vi "质控数据存储(子VI).vi"(4 "CODMn":refnum<vi>, 6 "总磷":refnum<vi>, 7 "CODCr":refnum<vi>, 10 "氨氮":refnum<vi>, 11 "总氮":refnum<vi>) -> ()   [LabVIEW 2016, in "质控单元.lvlib"]
uses:
  <vilib>/ptbypt/NI_PtbyPt.lvlib
panel:
  out "columns":string[](array[string])
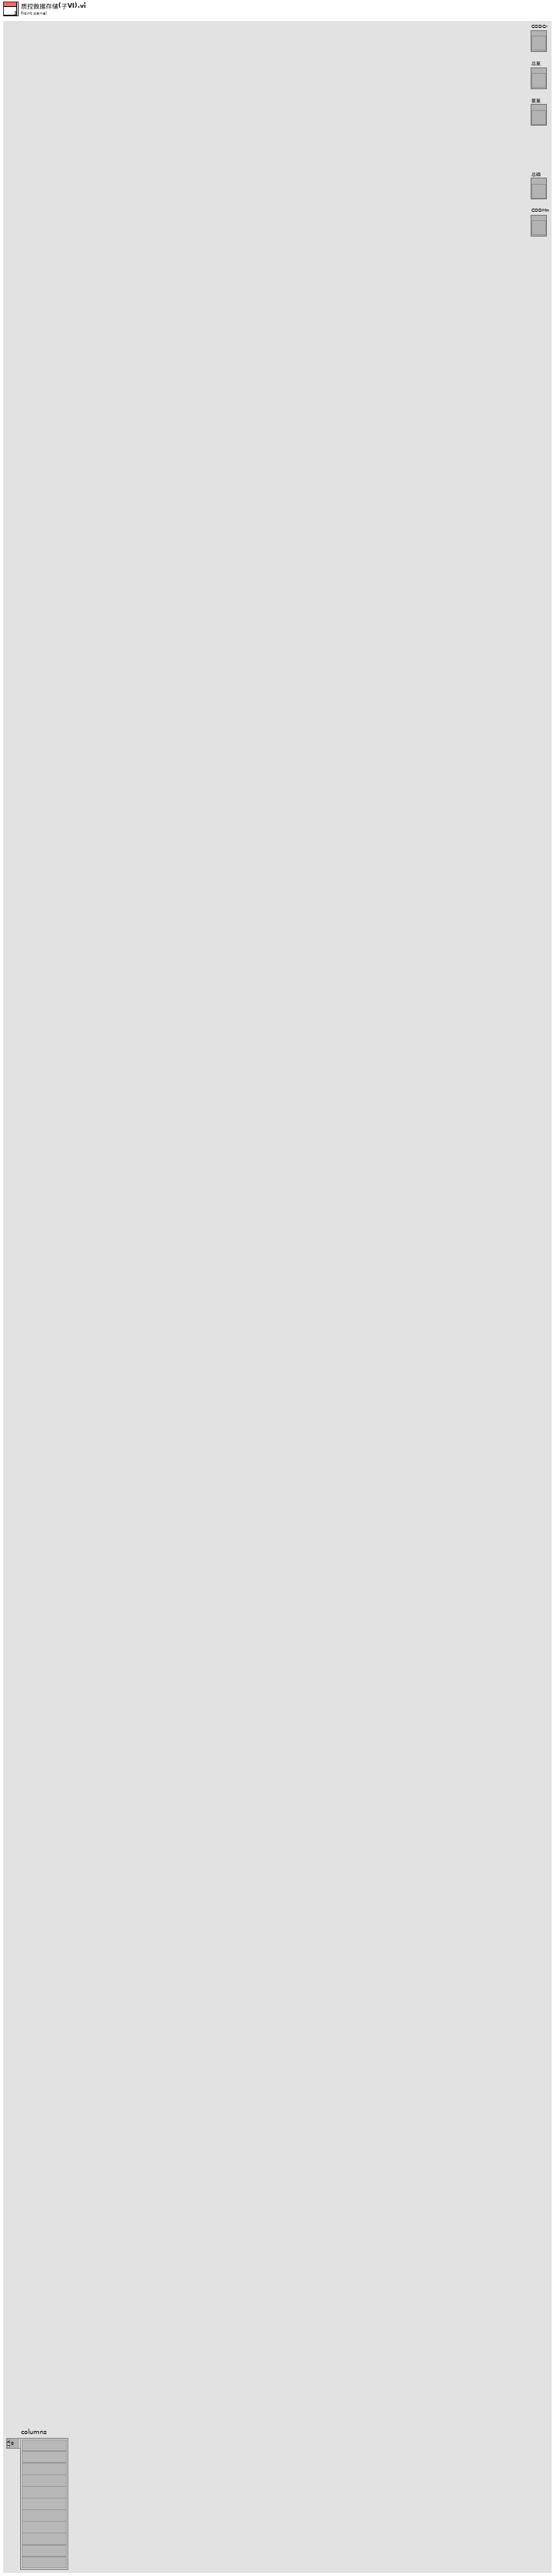
[diagram p1: front panel]
types:
  T1 = cluster{"时间":timestamp, "参数":string, "数据类型":string, "加标前水样测试时间":timestamp, "加标前水样浓度值（mg/L)":sgl, "加标后水样浓度值（mg/L)":sgl, "加标母液浓度值（mg/L)":sgl, "加标体积":dbl, "加标水杯定容体积":dbl, "加标回收率":dbl}
  T2 = cluster{"因子编码":u32, "单位":u16, "标样参考值":sgl, "水样数据时间":timestamp, "水样实测值":sgl, "水样数据标识":string, "标样数据时间":timestamp, "标样实测值":sgl, "标样数据标识":string, "空白数据时间":timestamp, "空白实测值":sgl, "空白数据标识":string, "零点核查数据时间":timestamp, "零点核查实测值":sgl, "零点核查数据标识":string, "跨度核查数据时间":timestamp, "跨度核查实测值":sgl, "跨度核查数据标识":string, "加标回收数据时间":timestamp, "加标回收实测值":sgl, "加标回收数据标识":string, "平行样数据时间":timestamp, "平行样实测值":sgl, "平行样数据标识":string}
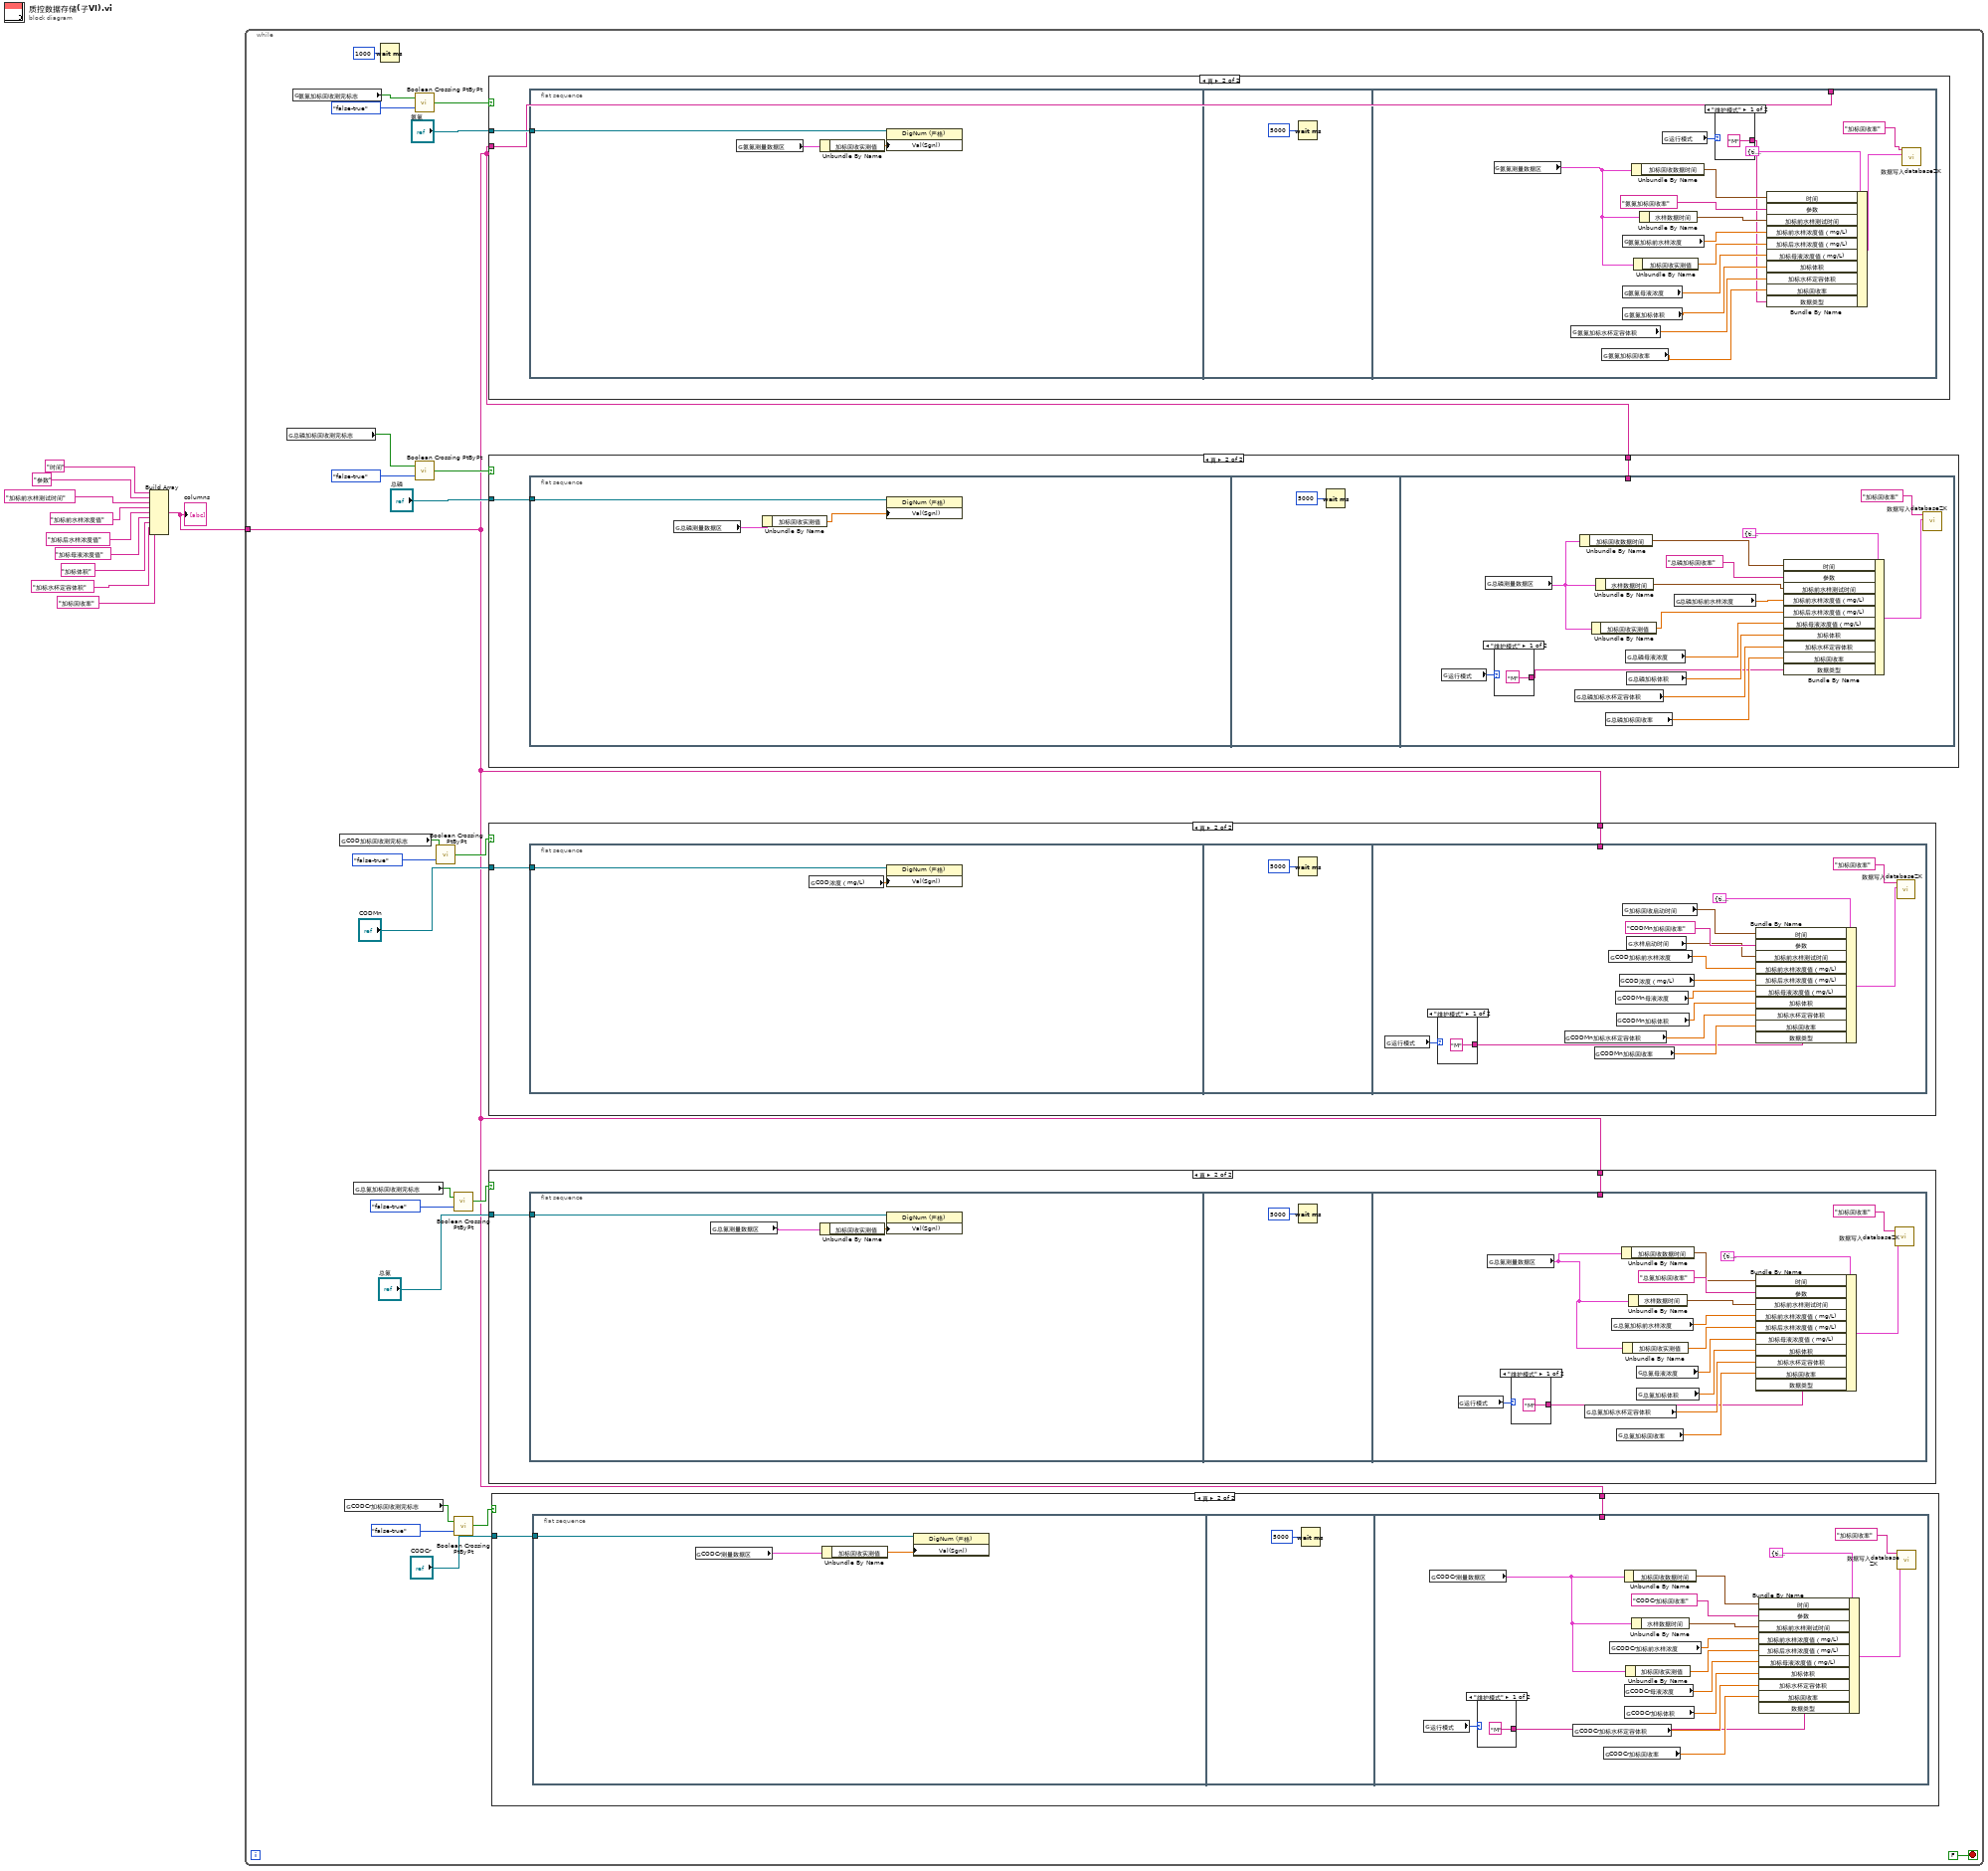
[diagram p0: block diagram]
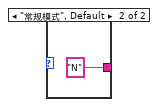
[diagram p3: hidden frame]
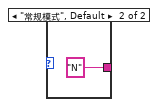
[diagram p5: hidden frame]
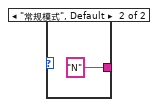
[diagram p7: hidden frame]
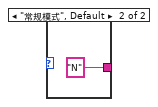
[diagram p9: hidden frame]
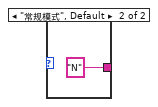
[diagram p11: hidden frame]
diagram:
  n1 = Build Array("时间" ("table"), "参数" ("table"), "加标前水样测试时间" ("table"), "加标前水样浓度值" ("元素"), "加标后水样浓度值" ("元素"), "加标母液浓度值" ("元素"), "加标体积" ("元素"), "加标水杯定容体积" ("元素"), "加标回收率" ("元素")) -> (w1:string[])
  "columns" <- w1
  n2 = while {
    tunnel: w1 -> [w11]
    stop <- FALSE stop-if-true
    n3 = global read "质控测完标志全局 1.vi" "总磷加标回收测完标志"() -> (w24:bool)
    n4 = global read "质控测完标志全局 1.vi" "氨氮加标回收测完标志"() -> (w19:bool)
    n5 = global read "质控测完标志全局 1.vi" "COD加标回收测完标志"() -> (w26:bool)
    n6 = global read "质控测完标志全局 1.vi" "CODCr加标回收测完标志"() -> (w32:bool)
    n7 = global read "质控测完标志全局 1.vi" "总氮加标回收测完标志"() -> (w29:bool)
    n8 = Wait (ms)(milliseconds to wait=u32 1000 ("等待时间（毫秒）")) -> ()  [unwired: 1 out]
    n9 = call <vilib>:"Boolean Crossing PtByPt.vi"("direction"=enum16{"either", "false-true", "true-false"}."false-true", "input"=w19) -> ("crossing"=w20:bool)  [unwired: 1 in]
    n10 = call <vilib>:"Boolean Crossing PtByPt.vi"("direction"=enum16{"either", "false-true", "true-false"}."false-true", "input"=w24) -> ("crossing"=w23:bool)  [unwired: 1 in]
    n11 = call <vilib>:"Boolean Crossing PtByPt.vi"("direction"=enum16{"either", "false-true", "true-false"}."false-true", "input"=w26) -> ("crossing"=w27:bool)  [unwired: 1 in]
    n12 = call <vilib>:"Boolean Crossing PtByPt.vi"("direction"=enum16{"either", "false-true", "true-false"}."false-true", "input"=w29) -> ("crossing"=w30:bool)  [unwired: 1 in]
    n13 = call <vilib>:"Boolean Crossing PtByPt.vi"("direction"=enum16{"either", "false-true", "true-false"}."false-true", "input"=w32) -> ("crossing"=w33:bool)  [unwired: 1 in]
    n14 = case shown="真" w20 {
      tunnel: "氨氮" -> [_ w125]
      tunnel: w11 -> [_ w124]
      frame False {
      }
      frame True {
        n15 = flat-sequence {
          tunnel: w125 -> [w126]
          tunnel: w124 -> [_]
          frame #0 {
            n16 = global read "与氨氮交互全局.vi" "氨氮测量数据区"() -> (w127:T2)
            n17 = Unbundle By Name(w127) -> ("加标回收实测值"=w128:sgl)
            n18 = property on="属性节点" class="DigNum (严格)"(reference=w126, "Val(Sgnl)"=w128) -> ()  [unwired: 1 in, 2 out]
          }
          frame #1 {
            n19 = Wait (ms)(milliseconds to wait=u32 5000 ("等待时间（毫秒）")) -> ()  [unwired: 1 out]
          }
          frame #2 {
            n20 = global read "与氨氮交互全局.vi" "氨氮测量数据区"() -> (w139:T2)
            n21 = global read "加标回收状态全局变量.vi" "氨氮加标水杯定容体积"() -> (w136:dbl)
            n22 = global read "加标回收状态全局变量.vi" "氨氮加标回收率"() -> (w137:dbl)
            n23 = global read "水样浓度全局.vi" "氨氮加标前水样浓度"() -> (w144:dbl)
            n24 = global read "加标回收状态全局变量.vi" "氨氮母液浓度"() -> (w134:dbl)
            n25 = global read "加标回收状态全局变量.vi" "氨氮加标体积"() -> (w135:dbl)
            n26 = Unbundle By Name(w139) -> ("加标回收数据时间"=w142:timestamp)
            n27 = Unbundle By Name(w139) -> ("加标回收实测值"=w143:sgl)
            n28 = Unbundle By Name(w139) -> ("水样数据时间"=w140:timestamp)
            n29 = global read "系统交互.vi" "运行模式"() -> (w131:enum16{"维护模式", "常规模式", "应急模式", "质控模式"})
            n30 = case shown="\"维护模式\"" w131 {
              tunnel: ["M" "N"] -> w130
              frame "维护模式" {
              }
              frame "常规模式", Default {
              }
            }
            n31 = Bundle By Name(cluster=T1 {"时间"=timestamp(0 s since 1904-01-01), "参数"="", "数据类型"="N", "加标前水样测试时间"=timestamp(0 s since 1904-01-01), "加标前水样浓度值（mg/L)"=0.0, "加标后水样浓度值（mg/L)"=0.0, "加标母液浓度值（mg/L)"=0.0, "加标体积"=0.0, "加标水杯定容体积"=0.0, "加标回收率"=0.0} ("data"), "时间"=w142, "参数"="氨氮加标回收率" ("table"), "加标前水样测试时间"=w140, "加标前水样浓度值（mg/L)"=w144, "加标后水样浓度值（mg/L)"=w143, "加标母液浓度值（mg/L)"=w134, "加标体积"=w135, "加标水杯定容体积"=w136, "加标回收率"=w137, "数据类型"=w130) -> (w132:T1)
            n32 = call "数据写入databaseZK.vi"("data"=w132, "table"="加标回收率") -> ()  [unwired: 9 in, 1 out]
          }
        }
      }
    }
    n33 = case shown="真" w23 {
      tunnel: "总磷" -> [_ w102]
      tunnel: w11 -> [_ w101]
      frame False {
      }
      frame True {
        n34 = flat-sequence {
          tunnel: w102 -> [w103]
          tunnel: w101 -> [_]
          frame #0 {
            n35 = global read "与总磷交互全局.vi" "总磷测量数据区"() -> (w104:T2)
            n36 = Unbundle By Name(w104) -> ("加标回收实测值"=w105:sgl)
            n37 = property on="属性节点" class="DigNum (严格)"(reference=w103, "Val(Sgnl)"=w105) -> ()  [unwired: 1 in, 2 out]
          }
          frame #1 {
            n38 = Wait (ms)(milliseconds to wait=u32 5000 ("等待时间（毫秒）")) -> ()  [unwired: 1 out]
          }
          frame #2 {
            n39 = global read "系统交互.vi" "运行模式"() -> (w108:enum16{"维护模式", "常规模式", "应急模式", "质控模式"})
            n40 = global read "与总磷交互全局.vi" "总磷测量数据区"() -> (w116:T2)
            n41 = case shown="\"维护模式\"" w108 {
              tunnel: ["M" "N"] -> w107
              frame "维护模式" {
              }
              frame "常规模式", Default {
              }
            }
            n42 = global read "加标回收状态全局变量.vi" "总磷加标水杯定容体积"() -> (w112:dbl)
            n43 = Unbundle By Name(w116) -> ("加标回收数据时间"=w119:timestamp)
            n44 = Unbundle By Name(w116) -> ("加标回收实测值"=w117:sgl)
            n45 = Unbundle By Name(w116) -> ("水样数据时间"=w118:timestamp)
            n46 = global read "加标回收状态全局变量.vi" "总磷加标回收率"() -> (w111:dbl)
            n47 = global read "加标回收状态全局变量.vi" "总磷母液浓度"() -> (w114:dbl)
            n48 = global read "加标回收状态全局变量.vi" "总磷加标体积"() -> (w113:dbl)
            n49 = global read "水样浓度全局.vi" "总磷加标前水样浓度"() -> (w121:dbl)
            n50 = Bundle By Name(cluster=T1 {"时间"=timestamp(0 s since 1904-01-01), "参数"="", "数据类型"="N", "加标前水样测试时间"=timestamp(0 s since 1904-01-01), "加标前水样浓度值（mg/L)"=0.0, "加标后水样浓度值（mg/L)"=0.0, "加标母液浓度值（mg/L)"=0.0, "加标体积"=0.0, "加标水杯定容体积"=0.0, "加标回收率"=0.0} ("data"), "时间"=w119, "参数"="总磷加标回收率" ("table"), "加标前水样测试时间"=w118, "加标前水样浓度值（mg/L)"=w121, "加标后水样浓度值（mg/L)"=w117, "加标母液浓度值（mg/L)"=w114, "加标体积"=w113, "加标水杯定容体积"=w112, "加标回收率"=w111, "数据类型"=w107) -> (w109:T1)
            n51 = call "数据写入databaseZK.vi"("data"=w109, "table"="加标回收率") -> ()  [unwired: 9 in, 1 out]
          }
        }
      }
    }
    n52 = case shown="真" w27 {
      tunnel: "CODMn" -> [_ w81]
      tunnel: w11 -> [_ w80]
      frame False {
      }
      frame True {
        n53 = flat-sequence {
          tunnel: w81 -> [w82]
          tunnel: w80 -> [_]
          frame #0 {
            n54 = global read "与CODMn交互全局.vi" "COD浓度（mg/L)"() -> (w83:dbl)
            n55 = property on="属性节点" class="DigNum (严格)"(reference=w82, "Val(Sgnl)"=w83) -> ()  [unwired: 1 in, 2 out]
          }
          frame #1 {
            n56 = Wait (ms)(milliseconds to wait=u32 5000 ("等待时间（毫秒）")) -> ()  [unwired: 1 out]
          }
          frame #2 {
            n57 = global read "系统交互.vi" "运行模式"() -> (w86:enum16{"维护模式", "常规模式", "应急模式", "质控模式"})
            n58 = case shown="\"维护模式\"" w86 {
              tunnel: ["M" "N"] -> w85
              frame "维护模式" {
              }
              frame "常规模式", Default {
              }
            }
            n59 = global read "加标回收状态全局变量.vi" "CODMn加标水杯定容体积"() -> (w90:dbl)
            n60 = global read "加标回收状态全局变量.vi" "CODMn加标回收率"() -> (w89:dbl)
            n61 = global read "水样浓度全局.vi" "COD加标前水样浓度"() -> (w98:dbl)
            n62 = global read "加标回收状态全局变量.vi" "CODMn母液浓度"() -> (w92:dbl)
            n63 = global read "加标回收状态全局变量.vi" "CODMn加标体积"() -> (w91:dbl)
            n64 = global read "与CODMn交互全局.vi" "COD浓度（mg/L)"() -> (w97:dbl)
            n65 = global read "与CODMn交互全局.vi" "加标回收启动时间"() -> (w95:timestamp)
            n66 = global read "与CODMn交互全局.vi" "水样启动时间"() -> (w94:timestamp)
            n67 = Bundle By Name(cluster=T1 {"时间"=timestamp(0 s since 1904-01-01), "参数"="", "数据类型"="N", "加标前水样测试时间"=timestamp(0 s since 1904-01-01), "加标前水样浓度值（mg/L)"=0.0, "加标后水样浓度值（mg/L)"=0.0, "加标母液浓度值（mg/L)"=0.0, "加标体积"=0.0, "加标水杯定容体积"=0.0, "加标回收率"=0.0} ("data"), "时间"=w95, "参数"="CODMn加标回收率" ("table"), "加标前水样测试时间"=w94, "加标前水样浓度值（mg/L)"=w98, "加标后水样浓度值（mg/L)"=w97, "加标母液浓度值（mg/L)"=w92, "加标体积"=w91, "加标水杯定容体积"=w90, "加标回收率"=w89, "数据类型"=w85) -> (w87:T1)
            n68 = call "数据写入databaseZK.vi"("data"=w87, "table"="加标回收率") -> ()  [unwired: 9 in, 1 out]
          }
        }
      }
    }
    n69 = case shown="真" w30 {
      tunnel: "总氮" -> [_ w58]
      tunnel: w11 -> [_ w57]
      frame False {
      }
      frame True {
        n70 = flat-sequence {
          tunnel: w58 -> [w59]
          tunnel: w57 -> [_]
          frame #0 {
            n71 = global read "与总氮交互全局.vi" "总氮测量数据区"() -> (w60:T2)
            n72 = Unbundle By Name(w60) -> ("加标回收实测值"=w61:sgl)
            n73 = property on="属性节点" class="DigNum (严格)"(reference=w59, "Val(Sgnl)"=w61) -> ()  [unwired: 1 in, 2 out]
          }
          frame #1 {
            n74 = Wait (ms)(milliseconds to wait=u32 5000 ("等待时间（毫秒）")) -> ()  [unwired: 1 out]
          }
          frame #2 {
            n75 = global read "系统交互.vi" "运行模式"() -> (w64:enum16{"维护模式", "常规模式", "应急模式", "质控模式"})
            n76 = global read "与总氮交互全局.vi" "总氮测量数据区"() -> (w71:T2)
            n77 = case shown="\"维护模式\"" w64 {
              tunnel: ["M" "N"] -> w63
              frame "维护模式" {
              }
              frame "常规模式", Default {
              }
            }
            n78 = global read "加标回收状态全局变量.vi" "总氮加标水杯定容体积"() -> (w68:dbl)
            n79 = global read "水样浓度全局.vi" "总氮加标前水样浓度"() -> (w77:dbl)
            n80 = global read "加标回收状态全局变量.vi" "总氮加标回收率"() -> (w67:dbl)
            n81 = Unbundle By Name(w71) -> ("加标回收数据时间"=w74:timestamp)
            n82 = Unbundle By Name(w71) -> ("加标回收实测值"=w76:sgl)
            n83 = Unbundle By Name(w71) -> ("水样数据时间"=w73:timestamp)
            n84 = global read "加标回收状态全局变量.vi" "总氮母液浓度"() -> (w70:dbl)
            n85 = global read "加标回收状态全局变量.vi" "总氮加标体积"() -> (w69:dbl)
            n86 = Bundle By Name(cluster=T1 {"时间"=timestamp(0 s since 1904-01-01), "参数"="", "数据类型"="N", "加标前水样测试时间"=timestamp(0 s since 1904-01-01), "加标前水样浓度值（mg/L)"=0.0, "加标后水样浓度值（mg/L)"=0.0, "加标母液浓度值（mg/L)"=0.0, "加标体积"=0.0, "加标水杯定容体积"=0.0, "加标回收率"=0.0} ("data"), "时间"=w74, "参数"="总氮加标回收率" ("table"), "加标前水样测试时间"=w73, "加标前水样浓度值（mg/L)"=w77, "加标后水样浓度值（mg/L)"=w76, "加标母液浓度值（mg/L)"=w70, "加标体积"=w69, "加标水杯定容体积"=w68, "加标回收率"=w67, "数据类型"=w63) -> (w65:T1)
            n87 = call "数据写入databaseZK.vi"("data"=w65, "table"="加标回收率") -> ()  [unwired: 9 in, 1 out]
          }
        }
      }
    }
    n88 = case shown="真" w33 {
      tunnel: "CODCr" -> [_ w35]
      tunnel: w11 -> [_ w34]
      frame False {
      }
      frame True {
        n89 = flat-sequence {
          tunnel: w35 -> [w36]
          tunnel: w34 -> [_]
          frame #0 {
            n90 = global read "与CODCr交互全局.vi" "CODCr测量数据区"() -> (w38:T2)
            n91 = Unbundle By Name(w38) -> ("加标回收实测值"=w37:sgl)
            n92 = property on="属性节点" class="DigNum (严格)"(reference=w36, "Val(Sgnl)"=w37) -> ()  [unwired: 1 in, 2 out]
          }
          frame #1 {
            n93 = Wait (ms)(milliseconds to wait=u32 5000 ("等待时间（毫秒）")) -> ()  [unwired: 1 out]
          }
          frame #2 {
            n94 = global read "系统交互.vi" "运行模式"() -> (w41:enum16{"维护模式", "常规模式", "应急模式", "质控模式"})
            n95 = global read "与CODCr交互全局.vi" "CODCr测量数据区"() -> (w48:T2)
            n96 = case shown="\"维护模式\"" w41 {
              tunnel: ["M" "N"] -> w40
              frame "维护模式" {
              }
              frame "常规模式", Default {
              }
            }
            n97 = global read "加标回收状态全局变量.vi" "CODCr加标水杯定容体积"() -> (w45:dbl)
            n98 = global read "加标回收状态全局变量.vi" "CODCr加标回收率"() -> (w44:dbl)
            n99 = global read "水样浓度全局.vi" "CODCr加标前水样浓度"() -> (w54:dbl)
            n100 = Unbundle By Name(w48) -> ("加标回收数据时间"=w51:timestamp)
            n101 = global read "加标回收状态全局变量.vi" "CODCr母液浓度"() -> (w47:dbl)
            n102 = global read "加标回收状态全局变量.vi" "CODCr加标体积"() -> (w46:dbl)
            n103 = Unbundle By Name(w48) -> ("加标回收实测值"=w53:sgl)
            n104 = Unbundle By Name(w48) -> ("水样数据时间"=w50:timestamp)
            n105 = Bundle By Name(cluster=T1 {"时间"=timestamp(0 s since 1904-01-01), "参数"="", "数据类型"="N", "加标前水样测试时间"=timestamp(0 s since 1904-01-01), "加标前水样浓度值（mg/L)"=0.0, "加标后水样浓度值（mg/L)"=0.0, "加标母液浓度值（mg/L)"=0.0, "加标体积"=0.0, "加标水杯定容体积"=0.0, "加标回收率"=0.0} ("data"), "时间"=w51, "参数"="CODCr加标回收率" ("table"), "加标前水样测试时间"=w50, "加标前水样浓度值（mg/L)"=w54, "加标后水样浓度值（mg/L)"=w53, "加标母液浓度值（mg/L)"=w47, "加标体积"=w46, "加标水杯定容体积"=w45, "加标回收率"=w44, "数据类型"=w40) -> (w42:T1)
            n106 = call "数据写入databaseZK.vi"("data"=w42, "table"="加标回收率") -> ()  [unwired: 9 in, 1 out]
          }
        }
      }
    }
  }
